vi "RVC To Polar.vi"(7 "initialize?":bool, 10 "pose":dbl[](array[numeric])=[5.0, 5.0, 0.0], 11 "desired pose":dbl[](array[numeric])=[5.0, 5.0, 0.0]) -> (0 "direction":dbl, 1 "beta":dbl, 2 "alpha":dbl, 3 "rho":dbl)   [LabVIEW 2017]
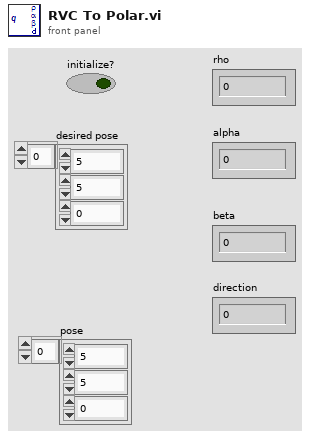
[diagram p1: front panel]
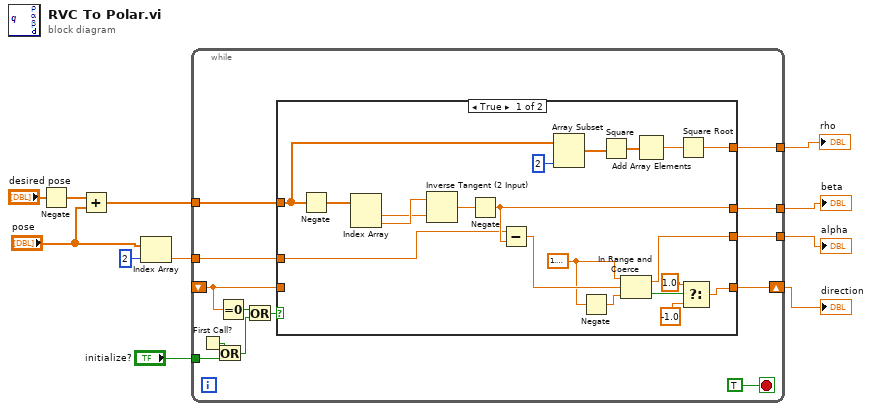
[diagram p0: block diagram]
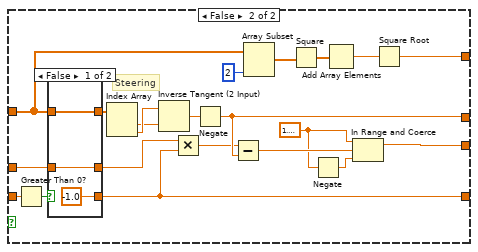
[diagram p2: hidden frame]
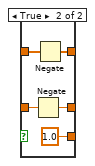
[diagram p3: hidden frame]
diagram:
  n1 = Negate(x="desired pose") -> (-x=w1:dbl[])
  n2 = Add(x=w1, y="pose") -> (x+y=w3:dbl[])
  n3 = Index Array(array="pose", index=2) -> (element=w4:dbl)
  n4 = while {
    shift-right: [w21] -> w9
    shift-left: _ -> [w18]
    tunnel: w3 -> [w23]
    tunnel: [w20] -> w11
    tunnel: [w22] -> w10
    tunnel: [w15] -> w8
    tunnel: "initialize?" -> [w13]
    tunnel: w4 -> [w12]
    stop <- TRUE stop-if-true
    n5 = First Call?() -> (First Call?: T/F=w24:bool)
    n6 = Or(x=w24, y=w13) -> (x .or. y?=w14:bool)
    n7 = Equal To 0?(x=w18) -> (x = 0?=w17:bool)
    n8 = Or(x=w17, y=w14) -> (x .or. y?=w19:bool)
    n9 = case shown="True" w19 {
      tunnel: w23 -> [w31 w51]
      tunnel: [w34 w58] -> w20
      tunnel: [w33 w56] -> w22
      tunnel: [w35 w47] -> w21
      tunnel: w18 -> [_ w57]
      tunnel: [w27 w48] -> w15
      tunnel: w12 -> [w25 w46]
      frame True {
        w40 = 1.5707963267948966
        n10 = Negate(x=w31) -> (-x=w26:dbl[])
        n11 = Index Array(array=w26) -> (element #1=w43:dbl, element #2=w44:dbl)  [unwired: 2 in]
        n12 = Inverse Tangent (2 Input)(1:w43, 2:w44) -> (0:w42:dbl)
        n13 = Negate(x=w42) -> (-x=w34:dbl)
        n14 = Subtract(x=w25, y=w34) -> (x-y=w41:dbl)
        n15 = Array Subset(array=w31, length=2) -> (w30:dbl[])  [unwired: 1 in]
        n16 = Negate(x=w40) -> (-x=w39:dbl)
        n17 = Square(x=w30) -> (x^2=w29:dbl[])
        n18 = In Range and Coerce(upper limit=w40, x=w41, lower limit=w39) -> (coerced(x)=w33:dbl, In Range?=w38:bool)
        n19 = Add Array Elements(numeric array=w29) -> (sum=w28:dbl)
        n20 = Square Root(x=w28) -> (sqrt(x)=w27:dbl)
        n21 = Select(t=1.0, s=w38, f=-1.0 ("t")) -> (s? t:f=w35:dbl)
      }
      frame False {
        w60 = 1.5707963267948966
        # "Steering"
        n22 = Greater Than 0?(x=w57) -> (x > 0?=w55:bool)
        n23 = case shown="False" w55 {
          tunnel: w51 -> [w67 w72]
          tunnel: [w67 w71] -> w63
          tunnel: [-1.0 ("t") 1.0 ("t")] -> w47
          tunnel: [w66 w69] -> w45
          tunnel: w46 -> [w66 w70]
          frame False {
          }
          frame True {
            n24 = Negate(x=w70) -> (-x=w69:dbl)
            n25 = Negate(x=w72) -> (-x=w71:dbl[])
          }
        }
        n26 = Index Array(array=w63) -> (element #1=w64:dbl, element #2=w65:dbl)  [unwired: 2 in]
        n27 = Inverse Tangent (2 Input)(1:w64, 2:w65) -> (0:w62:dbl)
        n28 = Multiply(x=w45, y=w47) -> (x*y=w49:dbl)
        n29 = Negate(x=w62) -> (-x=w58:dbl)
        n30 = Subtract(x=w49, y=w58) -> (x-y=w61:dbl)
        n31 = Array Subset(array=w51, length=2) -> (w53:dbl[])  [unwired: 1 in]
        n32 = Square(x=w53) -> (x^2=w52:dbl[])
        n33 = Negate(x=w60) -> (-x=w59:dbl)
        n34 = Add Array Elements(numeric array=w52) -> (sum=w50:dbl)
        n35 = In Range and Coerce(upper limit=w60, x=w61, lower limit=w59) -> (coerced(x)=w56:dbl)  [unwired: 1 out]
        n36 = Square Root(x=w50) -> (sqrt(x)=w48:dbl)
      }
    }
  }
  "beta" <- w11
  "alpha" <- w10
  "direction" <- w9
  "rho" <- w8
